vi "cw_2_1.vi"() -> ()   [LabVIEW 2022 SP3]
uses:
  <vilib>/numeric/Random Number (Range) DBL.vi
panel:
  in  "noise amplitude":ext=0.5
  out "Waveform Chart":dbl(graph)
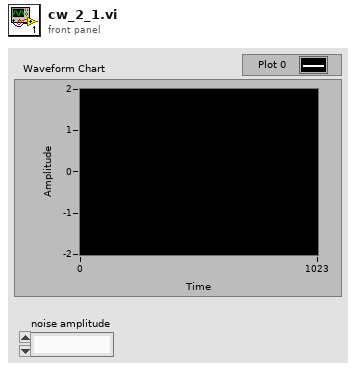
[diagram p1: front panel]
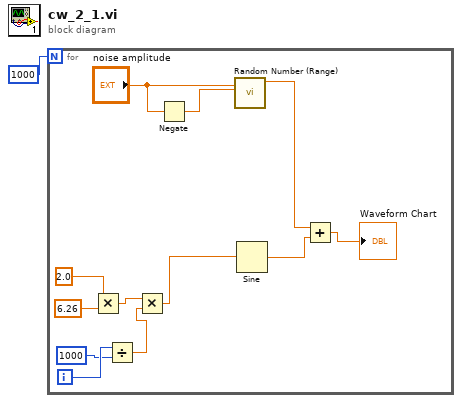
[diagram p0: block diagram]
diagram:
  n1 = for {
    N: 1000 -> [_]
    i -> [w12]
    n2 = Multiply(x=2.0, y=6.26) -> (x*y=w10:dbl)
    n3 = Divide(x=w12, y=1000) -> (x/y=w9:dbl)
    n4 = Multiply(x=w10, y=w9) -> (x*y=w8:dbl)
    n5 = Negate(x="noise amplitude") -> (-x=w3:ext)
    n6 = call-poly <vilib>:"Random Number (Range).vi"("lower bound (0)"=w3, "upper bound (100)"="noise amplitude") -> ("number"=w5:dbl)  [unwired: 9 in]
    n7 = Sine(x=w8) -> (sin(x)=w6:dbl)
    n8 = Add(x=w5, y=w6) -> (x+y=→"Waveform Chart":dbl)
  }
